vi "Reset Metodo.vi"(8 "error in (no error)":errorcluster, 11 "TektroniksTDS in":refnum<class "TektroniksTDS.lvclass">) -> (0 "error out":errorcluster, 3 "TektroniksTDS out":refnum<class "TektroniksTDS.lvclass">)   [LabVIEW 2020, in "TektroniksTDS.lvclass"]
uses:
  TektroniksTDS.lvclass
  TektroniksTDS.lvclass/TektroniksTDS.ctl
  <instrlib>/Tektronix TDS 200 1000 2000 Series/Tektronix TDS 200 1000 2000 Series.lvlib
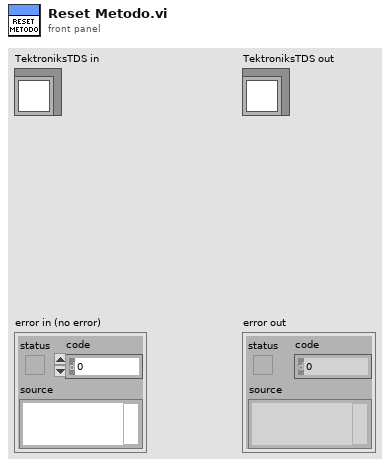
[diagram p1: front panel]
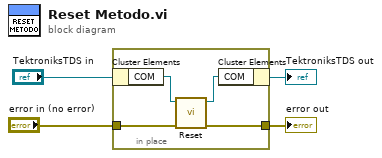
[diagram p0: block diagram]
diagram:
  n1 = in-place {
    in-place-border: "error in (no error)" -> [w8]
    in-place-border: [w5] -> w2
    n2 = in-place-cluster #1("TektroniksTDS in") -> ("COM"=w7:refnum<visa-resource-name>)
    n3 = call <instrlib>:"Reset.vi"("error in (no error)"=w8, "VISA resource name"=w7) -> ("error out"=w5:errorcluster, "VISA resource name out"=w6:refnum<visa-resource-name>)  [unwired: 8 in]
    n4 = in-place-cluster #1("COM"=w6) -> (→"TektroniksTDS out":refnum<class "TektroniksTDS.lvclass">)
  }
  "error out" <- w2
